vi "SetGXMLCfgTach.vi"(8 "error in (no error)":errorcluster, 10 "TachChanCfg":T1, 11 "Tachometer in":refnum<class "Tachometer.lvclass">) -> (0 "error out":errorcluster, 3 "Tachometer out":refnum<class "Tachometer.lvclass">)   [LabVIEW 2012, in "Measurement Channels.lvlib" / "Tachometer.lvclass"]
uses:
  Tachometer.lvclass
  TachProps_TD.ctl
  Tachometer.lvclass/Tachometer.ctl
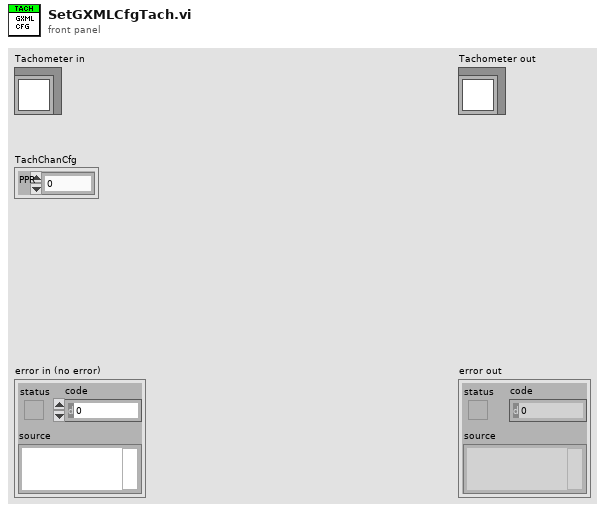
[diagram p1: front panel]
types:
  T1 = typedef "Measurement Channels.lvlib/Tachometer.lvclass/TachProps_TD.ctl" = cluster{"PPR":dbl}
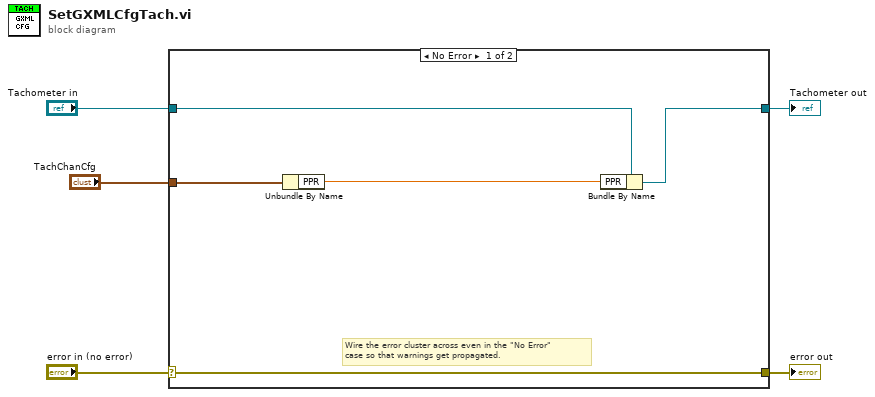
[diagram p0: block diagram]
diagram:
  n1 = case shown="No Error" "error in (no error)" {
    selector: "error in (no error)" -> [w10 w12]
    tunnel: [w10 w12] -> w4
    tunnel: [w6 w11] -> w2
    tunnel: "Tachometer in" -> [w7 w11]
    tunnel: "TachChanCfg" -> [w8 _]
    frame No Error {
      # "Wire the error cluster across even in the \"No Error\"\ncase so that warnings get propagated."
      n2 = Unbundle By Name(w8) -> ("PPR"=w9:dbl)
      n3 = Bundle By Name(cluster=w7, "PPR"=w9) -> (w6:refnum<class "Tachometer.lvclass">)
    }
    frame Error {
    }
  }
  "error out" <- w4
  "Tachometer out" <- w2
